vi "ZUP Initialize ADDRESS.vi"(8 "error in":errorcluster, 10 "ADDRESS":i16=1, 11 "VISA resource name":refnum<visa-resource-name>) -> (0 "error out":errorcluster, 3 "VISA resource name out":refnum<visa-resource-name>)   [LabVIEW 2012]
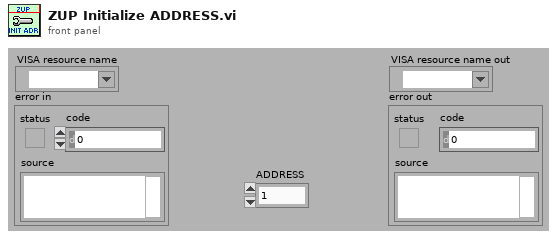
[diagram p1: front panel]
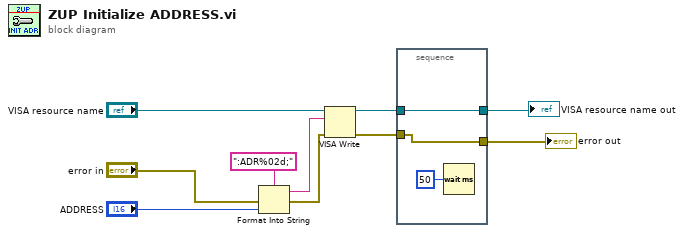
[diagram p0: block diagram]
diagram:
  n1 = Format Into String(format string=":ADR%02d;", error in="error in", "ADDRESS") -> (resulting string=w9:string, error out=w8:errorcluster)  [unwired: 1 in]
  n2 = VISA Write(VISA resource name="VISA resource name", write buffer=w9, error in (no error)=w8) -> (VISA resource name out=w4:refnum<visa-resource-name>, error out=w2:errorcluster)  [unwired: 1 out]
  n3 = stacked-sequence {
    tunnel: w4 -> [w13]
    tunnel: [w13] -> w3
    tunnel: w2 -> [w12]
    tunnel: [w12] -> w1
    frame #0 {
      n4 = Wait (ms)(milliseconds to wait=u32 50) -> ()  [unwired: 1 out]
    }
  }
  "VISA resource name out" <- w3
  "error out" <- w1
